vi "CropMelody (SubVI).vi"(10 "Array in":dbl[][](array[numeric]), 11 "Digital in":refnum<vi>) -> (3 "Array out":dbl[][](array[numeric]))   [LabVIEW 2014]
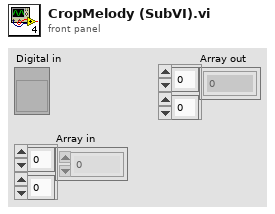
[diagram p1: front panel]
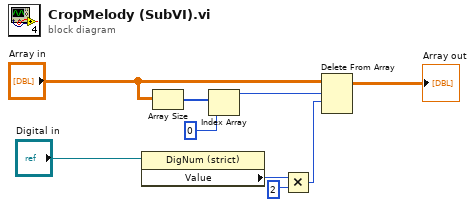
[diagram p0: block diagram]
diagram:
  n1 = property class="DigNum (strict)"(reference="Digital in") -> ("Value"=w6:i32)  [unwired: 1 in, 2 out]
  n2 = Array Size(array="Array in") -> (size(s)=w4:i32[])
  n3 = Index Array(array=w4, index=0) -> (element=w5:i32)
  n4 = Multiply(x=w6, y=2) -> (x*y=w9:i32)
  n5 = Delete From Array(array="Array in", length=w5, index (row)=w9) -> (array with subset deleted=→"Array out":dbl[][])  [unwired: 1 in, 1 out]
